vi "Main.vi"() -> ()   [LabVIEW 2019]
uses:
  Controls/#enum_DeliveryType.ctl
panel:
  in  "Stop":bool
  in  "Order Shipping":bool
  in  "Delivery Type":T1
  in  "Weight [kg]":dbl
  in  "Recipient's Address":string
  in  "Sender's Address":string
  in  "Recipient's Name:":string
  in  "Sender's Name:":string
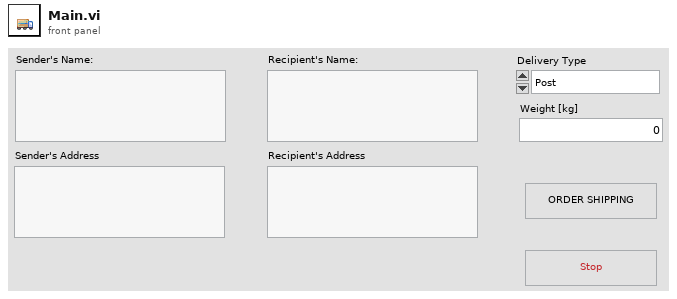
[diagram p1: front panel]
types:
  T1 = typedef "#enum_DeliveryType.ctl" = enum16{"Post", "Courier", "Pigeon"}
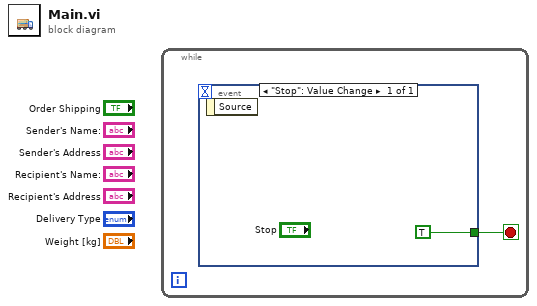
[diagram p0: block diagram]
diagram:
  n1 = while {
    stop <- w1 stop-if-true
    n2 = event shown="[0] \"Stop\": Value Change" {
      selector: _ -> [_]
      dyn-events: _ -> [_]
      timeout: _ -> [_]
      tunnel: [TRUE] -> w1
      event "Stop": Value Change {
        n3 = event-data() -> ()  [unwired: 1 in, 1 out]
      }
    }
  }
